vi "Get Minimum LabVIEW Version.vi"(8 "error in":errorcluster, 11 "9253 in":refnum<class "9253.lvclass">) -> (0 "error out":errorcluster, 2 "Minimum LabVIEW Version":i32, 3 "9253 out":refnum<class "9253.lvclass">)   [LabVIEW 2017, in "Modules.lvlib" / "9253.lvclass"]
uses:
  9253.lvclass
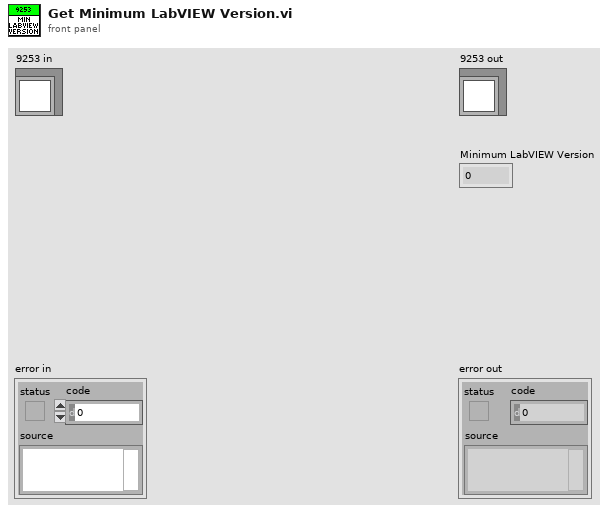
[diagram p1: front panel]
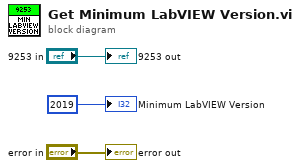
[diagram p0: block diagram]
diagram:
  "error out" <- "error in"
  "9253 out" <- "9253 in"
  "Minimum LabVIEW Version" <- 2019 ("Minimum LabVIEW Version")
